vi "networkstream_test_RIO.vi"() -> ()   [LabVIEW 2017]
panel:
  in  "stop":bool
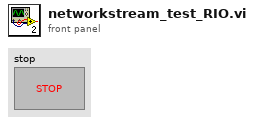
[diagram p1: front panel]
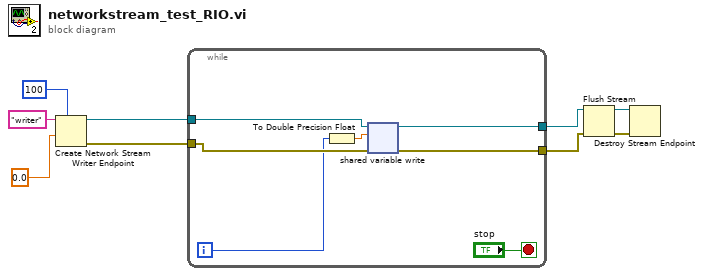
[diagram p0: block diagram]
diagram:
  n1 = Create Network Stream Writer Endpoint(7:100 ("writer buffer size"), 9:0.0, 11:"writer" ("writer name")) -> (0:w7:errorcluster, 3:w8:refnum<k21>)  [unwired: 4 in]
  n2 = while {
    tunnel: w8 -> [w15]
    tunnel: w7 -> [w14]
    tunnel: [w13] -> w2
    tunnel: [w12] -> w1
    i -> [w10]
    stop <- "stop" stop-if-true
    n3 = To Double Precision Float(number=w10) -> (double precision float=w11:dbl)
    n4 = shared-variable-write(w15, w14, w11) -> (w12:refnum<k21>, w13:errorcluster)  [unwired: 1 in, 1 out]
  }
  n5 = Flush Stream(8:w2, 11:w1) -> (0:w4:errorcluster, 3:w5:refnum<k21>)  [unwired: 2 in, 1 out]
  n6 = Destroy Stream Endpoint(8:w4, 11:w5) -> ()  [unwired: 1 out]
